vi "LimeLightData.vi"() -> ()   [LabVIEW 2019]
uses:
  <vilib>/Rock Robotics/Network Tables/NT Read Number.vi
  LabVIEW Data/Lime Light Test/Lime light global.vi
  <vilib>/Rock Robotics/Network Tables/NT Write Number.vi
panel:
  in  "Write Data Loop Time (ms)":u32
  in  "Read Data Loop Time (ms) (min 10)":u32
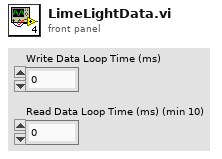
[diagram p1: front panel]
types:
  T1 = cluster{"offsetAngle H":dbl, "offsetAngle V":dbl, "area":dbl, "skew":dbl, "validTarget":dbl, "latency":dbl}
  T2 = typedef "WPI_DriverStationRobotMode2.ctl" = enum16{"Autonomous Disabled", "Autonomous Enabled", "Teleop Disabled", "Teleop Enabled", "Disconnected", "Finish", "Test Disabled", "Test Enabled", "Emergency Stopped"}
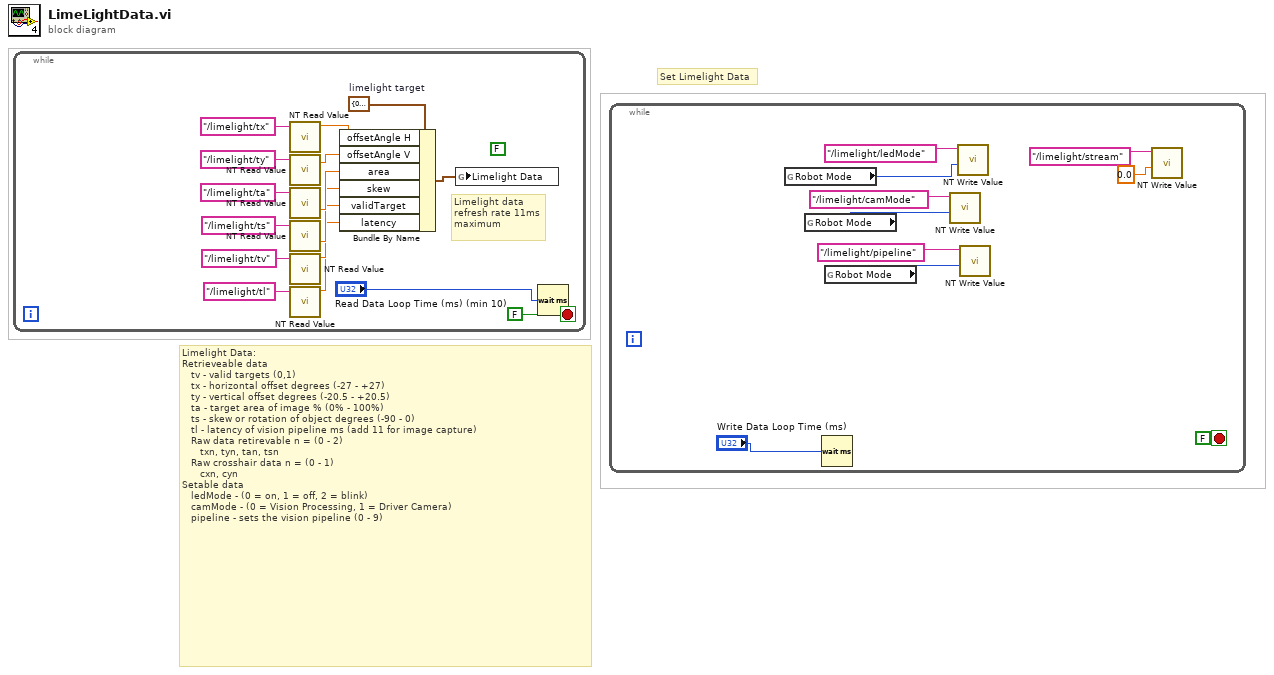
[diagram p0: block diagram]
diagram:
  # "Set Limelight Data"
  # "Limelight Data:\nRetrieveable data\n   tv - valid targets (0,1)\n   tx - horizontal offset degrees (-27 - +27)\n   ty - vertical offset degrees (-20.5 - +20.5)\n   ta - target area of image % (0% - 100%)\n   ts - skew or rotation of object degrees (-90 - 0)\n   tl - latency of vision pipeline ms (add 11 for image capture)\n   Raw data retirevable n = (0 - 2)\n      txn, tyn, tan, tsn\n   Raw crosshair data n = (0 - 1)\n      cxn, cyn\nSetable data\n   ledMode - (0 = on, 1 = off, 2 = blink)\n   camMode - (0 = Vision Processing, 1 = Driver Camera)\n   pipeline - sets the vision pipeline (0 - 9)"
  n1 = while {
    stop <- FALSE stop-if-true
    w12 = T1 {"offsetAngle H"=0.0, "offsetAngle V"=0.0, "area"=0.0, "skew"=0.0, "validTarget"=0.0, "latency"=0.0}  # limelight target
    (unwired) FALSE
    # "Limelight data\nrefresh rate 11ms\nmaximum"
    n2 = call-poly <vilib>:"NT Read Value.vi"("Name"="/limelight/tx") -> ("Numeric"=w11:dbl)  [unwired: 9 in, 1 out]
    n3 = call-poly <vilib>:"NT Read Value.vi"("Name"="/limelight/ty") -> ("Numeric"=w10:dbl)  [unwired: 9 in, 1 out]
    n4 = call-poly <vilib>:"NT Read Value.vi"("Name"="/limelight/ta") -> ("Numeric"=w9:dbl)  [unwired: 9 in, 1 out]
    n5 = call-poly <vilib>:"NT Read Value.vi"("Name"="/limelight/ts") -> ("Numeric"=w8:dbl)  [unwired: 9 in, 1 out]
    n6 = call-poly <vilib>:"NT Read Value.vi"("Name"="/limelight/tv") -> ("Numeric"=w6:dbl)  [unwired: 9 in, 1 out]
    n7 = call-poly <vilib>:"NT Read Value.vi"("Name"="/limelight/tl") -> ("Numeric"=w4:dbl)  [unwired: 9 in, 1 out]
    n8 = Bundle By Name(cluster=w12, "offsetAngle H"=w11, "offsetAngle V"=w10, "area"=w9, "skew"=w8, "validTarget"=w6, "latency"=w4) -> (w2:T1)
    n9 = global write "Lime light global.vi" "Limelight Data"(w2) -> ()
    n10 = Wait (ms)(milliseconds to wait="Read Data Loop Time (ms) (min 10)") -> ()  [unwired: 1 out]
  }
  n11 = while {
    stop <- FALSE stop-if-true
    n12 = global read "Lime light global.vi" "Robot Mode"() -> (w19:T2)
    n13 = global read "Lime light global.vi" "Robot Mode"() -> (w18:T2)
    n14 = Wait (ms)(milliseconds to wait="Write Data Loop Time (ms)") -> ()  [unwired: 1 out]
    n15 = global read "Lime light global.vi" "Robot Mode"() -> (w17:T2)
    n16 = call-poly <vilib>:"NT Write Value.vi"("Numeric"=w18, "Name"="/limelight/camMode") -> ()  [unwired: 9 in, 1 out]
    n17 = call-poly <vilib>:"NT Write Value.vi"("Numeric"=w19, "Name"="/limelight/ledMode") -> ()  [unwired: 9 in, 1 out]
    n18 = call-poly <vilib>:"NT Write Value.vi"("Numeric"=w17, "Name"="/limelight/pipeline") -> ()  [unwired: 9 in, 1 out]
    n19 = call-poly <vilib>:"NT Write Value.vi"("Numeric"=0.0 ("y"), "Name"="/limelight/stream") -> ()  [unwired: 9 in, 1 out]
  }
